vi "Get Shutter Line.vi"(8 "error in (no error)":errorcluster, 10 "Shutter":T1=enum."Cy3 (532 nm)", 11 "Uniblitz Shutter in":refnum<class "Uniblitz Shutter.lvclass">) -> (0 "error out":errorcluster, 1 "Index":i32, 2 "DAQmx Channel":refnum<k21>, 3 "Uniblitz Shutter out":refnum<class "Uniblitz Shutter.lvclass">)   [LabVIEW 2015, in "Uniblitz Shutter.lvlib" / "Uniblitz Shutter.lvclass"]
uses:
  Uniblitz Shutter.lvclass
  Resources/Type Defs/Excitation.ctl
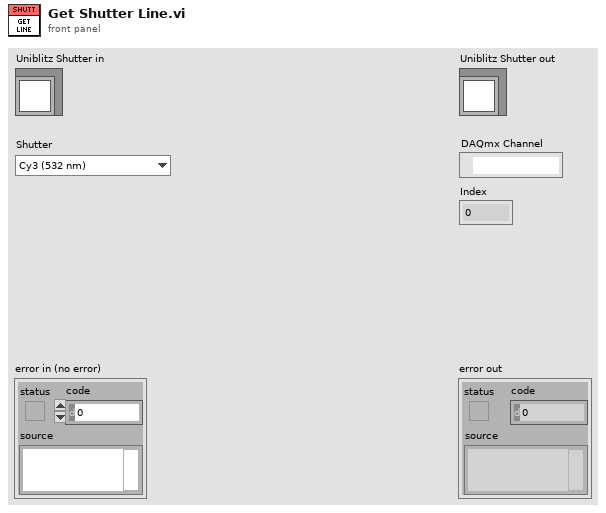
[diagram p1: front panel]
types:
  T1 = typedef "Excitation.ctl" = enum16{"Cy2 (473 nm)", "Cy3 (532 nm)", "Cy5 (639 nm)", "Cy7 (730 nm)"}
  T2 = cluster{"Excitation":T1, "DAQmx Channel":refnum<k21>, "Open?":bool}[]
  T3 = cluster{"Excitation":T1, "DAQmx Channel":refnum<k21>, "Open?":bool}
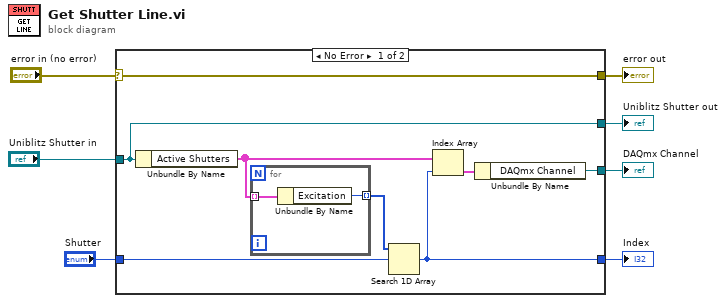
[diagram p0: block diagram]
diagram:
  n1 = case shown="No Error" "error in (no error)" {
    selector: "error in (no error)" -> [w15 w19]
    tunnel: [w15 w19] -> w6
    tunnel: [w11 w18] -> w4
    tunnel: "Uniblitz Shutter in" -> [w11 w18]
    tunnel: "Shutter" -> [w10 _]
    tunnel: [w9 _] -> w2
    tunnel: [w8 _] -> w1
    frame No Error {
      n2 = Unbundle By Name(w11) -> ("Active Shutters"=w13:T2)
      n3 = for {
        tunnel: w13 -> [w17] mode=indexing
        tunnel: [w16] -> w14 mode=indexing
        n4 = Unbundle By Name(w17) -> ("Excitation"=w16:T1)
      }
      n5 = Search 1D Array(1D array=w14, element=w10) -> (index of element=w8:i32)  [unwired: 1 in]
      n6 = Index Array(array=w13, index=w8) -> (element=w12:T3)
      n7 = Unbundle By Name(w12) -> ("DAQmx Channel"=w9:refnum<k21>)
    }
    frame Error {
    }
  }
  "error out" <- w6
  "Uniblitz Shutter out" <- w4
  "DAQmx Channel" <- w2
  "Index" <- w1
